vi "Configure RJDJ Extraction.vi"(0 "VISA resource name":refnum<visa-resource-name>, 1 "Enable RJDJ Measurement (T: Enable)":bool=TRUE, 2 "BER Level (6: 1E-12)":i32(ring)=6 items=["1E-6", "1E-7", "1E-8", "1E-9", "1E-10", "1E-11", "1E-12", "1E-13", "1E-14", "1E-15", "1E-16", "1E-17", "1E-18", "2.5E-3", "2.5E-10"], 5 "Measurement Source (1: Channel 1)":u16(ring)=1 items=["Channel 1"=1, "Channel 2"=2, "Channel 3"=3, "Channel 4"=4, "Function 1"=5, "Function 2"=6, "Function 3"=7, "Function 4"=8, "Memory 1"=9, "Memory 2"=10, "Memory 3"=11, "Memory 4"=12, "Differential 1"=61, "Differential 2"=62, "Common 1"=71, "Common 2"=72, "Clock"=15, "MTrend"=16, "MSpectrum"=17, "Equalized"=18], 7 "Bandwidth (0: Narrow)":i32(ring) items=["Narrow (Pink)", "Wide (White)"], 9 "Edge (2: Both)":i32(ring)=2 items=["Rising", "Falling ", "Both"], 11 "error in (no error)":errorcluster, 12 "Interpolation Mode (0: None)":i32(ring) items=["None", "Linear"], 13 "Measurement Units (0: Second)":i32(ring) items=["Second", "Unit Interval"], 14 "Pattern Length":T1={"ISI Filter Lead (-2)"=-2.0, "ISI Filter Lag (5)"=5.0, "Pattern Length Type (0: Periodic)"=0, "Number of Bits"=2000} {"Pattern Length Type (0: Periodic)" items=["Periodic", "Periodic (Number of Bits)", "Arbitrary"]}) -> (4 "VISA resource name out":refnum<visa-resource-name>, 15 "error out":errorcluster)   [LabVIEW 2013, in "Agilent 90000 Series.lvlib"]
doc: "Configures the RJDJ extraction measurement and its parameters. Calling this VI enables the RJDJ extraction measurement on the selected channel."
uses:
  Agilent 90000 Series.lvlib
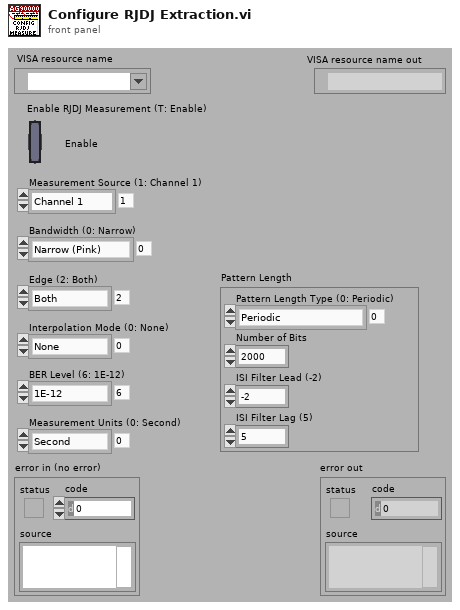
[diagram p1: front panel]
types:
  T1 = cluster{"ISI Filter Lead (-2)":dbl, "ISI Filter Lag (5)":dbl, "Pattern Length Type (0: Periodic)":i32, "Number of Bits":i32}
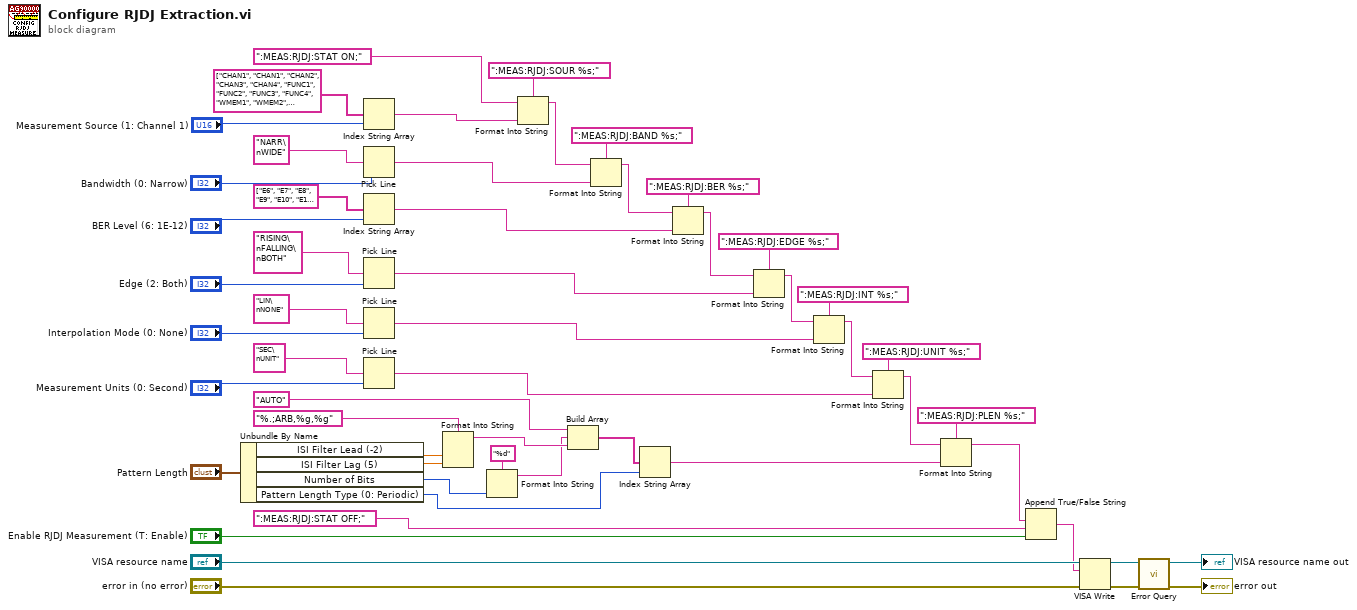
[diagram p0: block diagram]
diagram:
  n1 = Unbundle By Name("Pattern Length") -> ("ISI Filter Lead (-2)"=w41:dbl, "ISI Filter Lag (5)"=w40:dbl, "Number of Bits"=w32:i32, "Pattern Length Type (0: Periodic)"=w29:i32)
  n2 = Index String Array(1:"Measurement Source (1: Channel 1)", 2:string[] ["CHAN1", "CHAN1", "CHAN2", "CHAN3", "CHAN4", "FUNC1", "FUNC2", "FUNC3", "FUNC4", "WMEM1", "WMEM2", "WMEM3", "WMEM4", "AUX", "LINE", "CLOC", "MTR", "MSP", "EQU", "NONE", "DIG0", "DIG1", "DIG2", "DIG3", "DIG4", "DIG5", "DIG6", "DIG7", "DIG8", "DIG9", "DIG10", "DIG11", "DIG12", "DIG13", "DIG14", "DIG15", "", "", "", "", "", "POD1", "POD2", "", "", "", "", "", "", "", "", "BUS1", "BUS2", "BUS3", "BUS4", "", "", "", "", "", "", "DIFF1", "DIFF2", "", "", "", "", "", "", "", "", "COMM3", "COMM4"]) -> (0:w24:string)  [unwired: 1 out]
  n3 = Pick Line(multi-line string="NARR\nWIDE", line index="Bandwidth (0: Narrow)") -> (output string=w20:string)  [unwired: 1 out]
  n4 = Index String Array(1:"BER Level (6: 1E-12)", 2:string[] ["E6", "E7", "E8", "E9", "E10", "E11", "E12", "E13", "E14", "E15", "E16", "E17", "E18", "J2", "J9"]) -> (0:w17:string)  [unwired: 1 out]
  n5 = Pick Line(multi-line string="RISING\nFALLING\nBOTH", line index="Edge (2: Both)") -> (output string=w14:string)  [unwired: 1 out]
  n6 = Pick Line(multi-line string="LIN\nNONE", line index="Interpolation Mode (0: None)") -> (output string=w11:string)  [unwired: 1 out]
  n7 = Pick Line(multi-line string="SEC\nUNIT", line index="Measurement Units (0: Second)") -> (output string=w8:string)  [unwired: 1 out]
  n8 = Format Into String(format string="%.;ARB,%g,%g", w41, w40) -> (resulting string=w27:string)  [unwired: 2 in, 1 out]
  n9 = Format Into String(format string="%d", w32) -> (resulting string=w26:string)  [unwired: 2 in, 1 out]
  n10 = Format Into String(format string=":MEAS:RJDJ:SOUR %s;", initial string=":MEAS:RJDJ:STAT ON;" ("true string"), w24) -> (resulting string=w21:string)  [unwired: 1 in, 1 out]
  n11 = Build Array("AUTO" ("format string"), w26, w27) -> (w28:string[])
  n12 = Format Into String(format string=":MEAS:RJDJ:BAND %s;", initial string=w21, w20) -> (resulting string=w18:string)  [unwired: 1 in, 1 out]
  n13 = Index String Array(1:w29, 2:w28) -> (0:w5:string)  [unwired: 1 out]
  n14 = Format Into String(format string=":MEAS:RJDJ:BER %s;", initial string=w18, w17) -> (resulting string=w15:string)  [unwired: 1 in, 1 out]
  n15 = Format Into String(format string=":MEAS:RJDJ:EDGE %s;", initial string=w15, w14) -> (resulting string=w12:string)  [unwired: 1 in, 1 out]
  n16 = Format Into String(format string=":MEAS:RJDJ:INT %s;", initial string=w12, w11) -> (resulting string=w9:string)  [unwired: 1 in, 1 out]
  n17 = Format Into String(format string=":MEAS:RJDJ:UNIT %s;", initial string=w9, w8) -> (resulting string=w7:string)  [unwired: 1 in, 1 out]
  n18 = Format Into String(format string=":MEAS:RJDJ:PLEN %s;", initial string=w7, w5) -> (resulting string=w4:string)  [unwired: 1 in, 1 out]
  n19 = Append True/False String(1:"Enable RJDJ Measurement (T: Enable)", 2:":MEAS:RJDJ:STAT OFF;" ("false string"), 3:w4) -> (0:w3:string)  [unwired: 1 out]
  n20 = VISA Write(VISA resource name="VISA resource name", write buffer=w3, error in (no error)="error in (no error)") -> (VISA resource name out=w37:refnum<visa-resource-name>, error out=w34:errorcluster)  [unwired: 1 out]
  n21 = call "Error Query.vi"("error in (no error)"=w34, "VISA resource name"=w37) -> ("error out"=→"error out":errorcluster, "VISA resource name out"=→"VISA resource name out":refnum<visa-resource-name>)  [unwired: 8 out]
